vi "PhaseShifter demo close.vi"(8 "Error In":errorcluster, 10 "Toggle 6.lvclass":refnum<class "Toggle 6.lvclass">, 11 "Vector Network Analyzer.lvclass":refnum<class "Vector Network Analyzer.lvclass">) -> (0 "Error Out":errorcluster)   [LabVIEW 2020]
uses:
  Instruments/Vector Network Analyzer/Vector Network Analyzer.lvclass
  Devices/Toggle 6/Toggle 6.lvclass
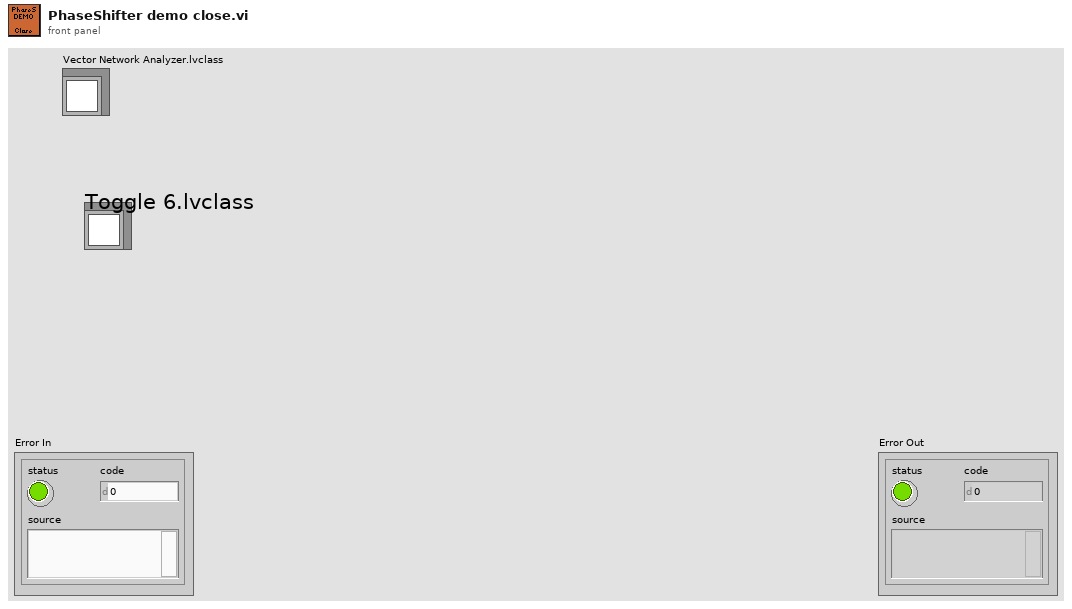
[diagram p1: front panel]
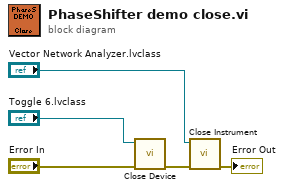
[diagram p0: block diagram]
diagram:
  n1 = call-dynamic "Close Device.vi"("error in (no error)"="Error In", "Device in"="Toggle 6.lvclass") -> ("error out"=w2:errorcluster)  [unwired: 8 in, 1 out]
  n2 = call-dynamic "Close Instrument.vi"("error in (no error)"=w2, "Instrument in"="Vector Network Analyzer.lvclass") -> ("error out"=→"Error Out":errorcluster)  [unwired: 8 in, 1 out]
